vi "LM_I_11.15 - Copy.vi"   [LabVIEW 2012]
uses:
  <vilib>/NXT/Block Support/NXT_MessageMailbox.ctl
  <vilib>/NXT/Subs/MotorOutput.ctl
  <vilib>/NXT/Block Support/NXT_InputPort.ctl
  <vilib>/NXT/Block Support/NXT_TimerIndex.ctl
  <vilib>/NXT/Block Support/NXT_OutputPort.ctl
  <vilib>/NXT/Dual Mode Library/Advanced/NXTFlag_Assign.vi
  <vilib>/NXT/Dual Mode Library/BT/BlueTooth_Write_String.vi
types:
  T1 = typedef "MotorOutput.ctl" = u8
  T2 = typedef "NXT_MessageMailbox.ctl" = u8
  T3 = typedef "LVHSConnector.ctl" = refnum<class "BrickReference.lvclass">
  T4 = typedef "NXT_InputPort.ctl" = u32
  T5 = typedef "NXT_TimerIndex.ctl" = u8
  T6 = typedef "NXT_OutputPort.ctl" = u8
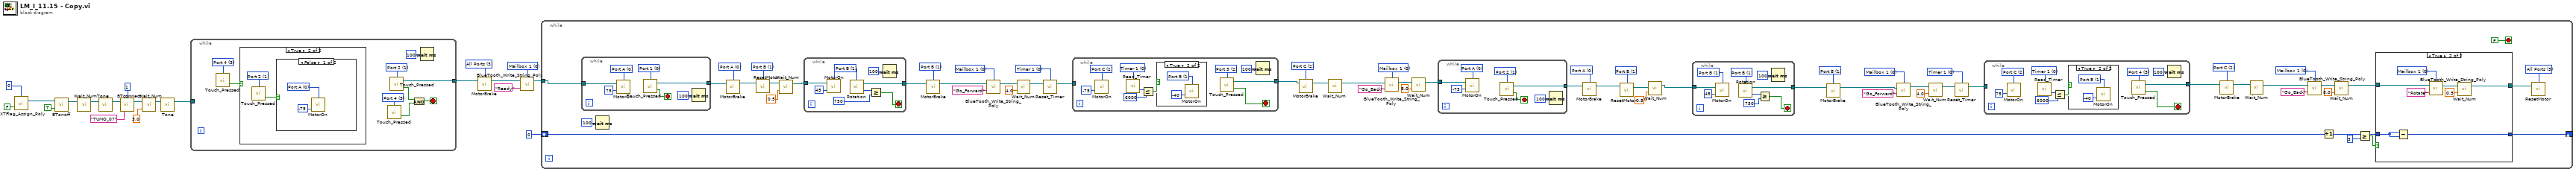
[diagram p0: block diagram]
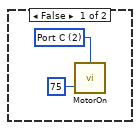
[diagram p2: hidden frame]
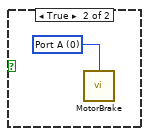
[diagram p3: hidden frame]
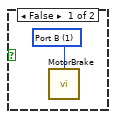
[diagram p4: hidden frame]
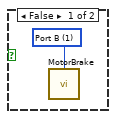
[diagram p6: hidden frame]
diagram:
  w7 = T1 3 items=["Port A"=0, "Port B"=1, "Port C"=2, "Ports A & B"=4, "Ports A & C"=5, "Ports B & C"=6, "All Ports"=3] ("Port (All Ports)")
  w8 = T2 0 items=["Mailbox 1", "Mailbox 2", "Mailbox 3", "Mailbox 4", "Mailbox 5", "Mailbox 6", "Mailbox 7", "Mailbox 8", "Mailbox 9", "Mailbox 10"] ("Mailbox")
  n1 = call-poly <vilib>:"NXTFlag_Assign_Poly.vi"("Flag State"=FALSE, "NXT/EV3 Flag Number"=i8 0) -> ("NXT/EV3"=w3:T3)  [unwired: 2 in]
  n2 = call <vilib>:"BTonoff.vi"("On/Off"=TRUE, "NXT/EV3"=w3) -> ("NXT/EV3"=w13:T3)  [unwired: 1 in, 1 out]
  n3 = call <vilib>:"Wait_Num.vi"("NXT/EV3"=w13) -> ("NXT/EV3"=w12:T3)  [unwired: 3 in]
  n4 = call <vilib>:"Tone.vi"("NXT/EV3"=w12) -> ("NXT/EV3"=w11:T3)  [unwired: 3 in]
  n5 = call <vilib>:"BTconnect.vi"("Partner Name"="TUMO_07", "NXT/EV3"=w11, "Connection"=u8 1) -> ("NXT/EV3"=w19:T3)  [unwired: 1 out]
  n6 = call <vilib>:"Wait_Num.vi"("Time (1 sec)"=sgl 3.0, "NXT/EV3"=w19) -> ("NXT/EV3"=w14:T3)  [unwired: 2 in]
  n7 = call <vilib>:"Tone.vi"("NXT/EV3"=w14) -> ("NXT/EV3"=w10:T3)  [unwired: 3 in]
  n8 = while {
    tunnel: w10 -> [_]
    tunnel: [w21] -> w5
    stop <- w25 stop-if-true
    w22 = T4 3 items=["Port 1", "Port 2", "Port 3", "Port 4"] ("Port (Port 1)")
    w27 = T4 3 items=["Port 1", "Port 2", "Port 3", "Port 4"] ("Port (Port 1)")
    w29 = T4 1 items=["Port 1", "Port 2", "Port 3", "Port 4"] ("Port (Port 1)")
    n9 = call <vilib>:"Touch_Pressed.vi"("Port (Port 1)"=w22) -> ("Yes / No"=w23:bool)  [unwired: 2 in, 1 out]
    n10 = case shown="True" w23 {
      frame False {
        w30 = T1 2 items=["Port A"=0, "Port B"=1, "Port C"=2, "Ports A & B"=4, "Ports A & C"=5, "Ports B & C"=6, "All Ports"=3] ("Output Port (All Ports)")
        n11 = call <vilib>:"MotorOn.vi"("Power (75)"=75, "Output Port (All Ports)"=w30) -> ()  [unwired: 2 in, 1 out]
      }
      frame True {
        w33 = T4 1 items=["Port 1", "Port 2", "Port 3", "Port 4"] ("Port (Port 1)")
        n12 = call <vilib>:"Touch_Pressed.vi"("Port (Port 1)"=w33) -> ("Yes / No"=w32:bool)  [unwired: 2 in, 1 out]
        n13 = case shown="False" w32 {
          frame False {
            w34 = T1 0 items=["Port A"=0, "Port B"=1, "Port C"=2, "Ports A & B"=4, "Ports A & C"=5, "Ports B & C"=6, "All Ports"=3] ("Output Port (All Ports)")
            n14 = call <vilib>:"MotorOn.vi"("Power (75)"=-75, "Output Port (All Ports)"=w34) -> ()  [unwired: 2 in, 1 out]
          }
          frame True {
            w36 = T1 0 items=["Port A"=0, "Port B"=1, "Port C"=2, "Ports A & B"=4, "Ports A & C"=5, "Ports B & C"=6, "All Ports"=3] ("Output Port (All Ports)")
            n15 = call <vilib>:"MotorBrake.vi"("Port (All Ports)"=w36) -> ()  [unwired: 3 in, 1 out]
          }
        }
      }
    }
    n16 = call <vilib>:"Touch_Pressed.vi"("Port (Port 1)"=w27) -> ("Yes / No"=w26:bool)  [unwired: 2 in, 1 out]
    n17 = call <vilib>:"Touch_Pressed.vi"("Port (Port 1)"=w29) -> ("Yes / No"=w28:bool, "NXT/EV3"=w21:T3)  [unwired: 2 in]
    n18 = And(x=w28, y=w26) -> (x .and. y?=w25:bool)
    n19 = Wait (ms)(milliseconds to wait=u32 100) -> ()  [unwired: 1 out]
  }
  n20 = call <vilib>:"MotorBrake.vi"("NXT/EV3"=w5, "Port (All Ports)"=w7) -> ("NXT/EV3"=w6:T3)  [unwired: 2 in]
  n21 = call-poly <vilib>:"BlueTooth_Write_String_Poly.vi"("Message"="Ready", "NXT/EV3"=w6, "Mailbox"=w8) -> ("NXT/EV3"=w4:T3)  [unwired: 1 in]
  n22 = while {
    shift-right: [w53] -> _
    shift-left: u32 0 ("milliseconds to wait") -> [w52]
    tunnel: w4 -> [w51]
    stop <- FALSE stop-if-true
    w37 = T1 3 items=["Port A"=0, "Port B"=1, "Port C"=2, "Ports A & B"=4, "Ports A & C"=5, "Ports B & C"=6, "All Ports"=3] ("Port (All Ports)")
    w43 = T5 0 items=["Timer 1", "Timer 2", "Timer 3"] ("Timer (Timer 1)")
    w47 = T5 0 items=["Timer 1", "Timer 2", "Timer 3"] ("Timer (Timer 1)")
    w91 = T1 1 items=["Port A"=0, "Port B"=1, "Port C"=2, "Ports A & B"=4, "Ports A & C"=5, "Ports B & C"=6, "All Ports"=3] ("Port (All Ports)")
    w90 = T1 1 items=["Port A"=0, "Port B"=1, "Port C"=2, "Ports A & B"=4, "Ports A & C"=5, "Ports B & C"=6, "All Ports"=3] ("Port (All Ports)")
    w76 = T2 0 items=["Mailbox 1", "Mailbox 2", "Mailbox 3", "Mailbox 4", "Mailbox 5", "Mailbox 6", "Mailbox 7", "Mailbox 8", "Mailbox 9", "Mailbox 10"] ("Mailbox")
    w74 = T2 0 items=["Mailbox 1", "Mailbox 2", "Mailbox 3", "Mailbox 4", "Mailbox 5", "Mailbox 6", "Mailbox 7", "Mailbox 8", "Mailbox 9", "Mailbox 10"] ("Mailbox")
    w69 = T2 0 items=["Mailbox 1", "Mailbox 2", "Mailbox 3", "Mailbox 4", "Mailbox 5", "Mailbox 6", "Mailbox 7", "Mailbox 8", "Mailbox 9", "Mailbox 10"] ("Mailbox")
    w67 = T1 2 items=["Port A"=0, "Port B"=1, "Port C"=2, "Ports A & B"=4, "Ports A & C"=5, "Ports B & C"=6, "All Ports"=3] ("Port (All Ports)")
    w65 = T1 0 items=["Port A"=0, "Port B"=1, "Port C"=2, "Ports A & B"=4, "Ports A & C"=5, "Ports B & C"=6, "All Ports"=3] ("Port (All Ports)")
    w64 = T1 2 items=["Port A"=0, "Port B"=1, "Port C"=2, "Ports A & B"=4, "Ports A & C"=5, "Ports B & C"=6, "All Ports"=3] ("Port (All Ports)")
    w61 = T1 1 items=["Port A"=0, "Port B"=1, "Port C"=2, "Ports A & B"=4, "Ports A & C"=5, "Ports B & C"=6, "All Ports"=3] ("Port (All Ports)")
    w60 = T1 0 items=["Port A"=0, "Port B"=1, "Port C"=2, "Ports A & B"=4, "Ports A & C"=5, "Ports B & C"=6, "All Ports"=3] ("Port (All Ports)")
    w57 = T2 0 items=["Mailbox 1", "Mailbox 2", "Mailbox 3", "Mailbox 4", "Mailbox 5", "Mailbox 6", "Mailbox 7", "Mailbox 8", "Mailbox 9", "Mailbox 10"] ("Mailbox")
    w55 = T1 1 items=["Port A"=0, "Port B"=1, "Port C"=2, "Ports A & B"=4, "Ports A & C"=5, "Ports B & C"=6, "All Ports"=3] ("Port (All Ports)")
    n23 = while {
      tunnel: [w160] -> w59
      tunnel: w51 -> [w159]
      stop <- w161 stop-if-true
      w162 = T4 0 items=["Port 1", "Port 2", "Port 3", "Port 4"] ("Port (Port 1)")
      w165 = T1 0 items=["Port A"=0, "Port B"=1, "Port C"=2, "Ports A & B"=4, "Ports A & C"=5, "Ports B & C"=6, "All Ports"=3] ("Output Port (All Ports)")
      n24 = call <vilib>:"MotorOn.vi"("Power (75)"=75, "NXT/EV3"=w159, "Output Port (All Ports)"=w165) -> ()  [unwired: 1 in, 1 out]
      n25 = call <vilib>:"Touch_Pressed.vi"("Port (Port 1)"=w162) -> ("Yes / No"=w161:bool, "NXT/EV3"=w160:T3)  [unwired: 2 in]
      n26 = Wait (ms)(milliseconds to wait=u32 100) -> ()  [unwired: 1 out]
    }
    n27 = Wait (ms)(milliseconds to wait=u32 100) -> ()  [unwired: 1 out]
    n28 = call <vilib>:"MotorBrake.vi"("NXT/EV3"=w59, "Port (All Ports)"=w60) -> ("NXT/EV3"=w58:T3)  [unwired: 2 in]
    n29 = call <vilib>:"ResetMotor.vi"("NXT/EV3"=w58, "Port (All Ports)"=w55) -> ("NXT/EV3"=w87:T3)  [unwired: 2 in]
    n30 = call <vilib>:"Wait_Num.vi"("Time (1 sec)"=sgl 0.5, "NXT/EV3"=w87) -> ("NXT/EV3"=w88:T3)  [unwired: 2 in]
    n31 = while {
      tunnel: w88 -> [w158]
      tunnel: [w152] -> w62
      stop <- w154 stop-if-true
      w156 = T1 1 items=["Port A"=0, "Port B"=1, "Port C"=2, "Ports A & B"=4, "Ports A & C"=5, "Ports B & C"=6, "All Ports"=3] ("Output Port (All Ports)")
      n32 = call <vilib>:"MotorOn.vi"("Power (75)"=45, "NXT/EV3"=w158, "Output Port (All Ports)"=w156) -> ()  [unwired: 1 in, 1 out]
      n33 = call <vilib>:"Rotation.vi"("Port (Port A)"=w156) -> ("Angle of Rotation"=w155:i32, "NXT/EV3"=w152:T3)  [unwired: 2 in]
      n34 = Greater Or Equal?(x=w155, y=750) -> (x >= y?=w154:bool)
      n35 = Wait (ms)(milliseconds to wait=u32 100) -> ()  [unwired: 1 out]
    }
    n36 = call <vilib>:"MotorBrake.vi"("NXT/EV3"=w62, "Port (All Ports)"=w61) -> ("NXT/EV3"=w63:T3)  [unwired: 2 in]
    n37 = call-poly <vilib>:"BlueTooth_Write_String_Poly.vi"("Message"="Go_Forward", "NXT/EV3"=w63, "Mailbox"=w57) -> ("NXT/EV3"=w50:T3)  [unwired: 1 in]
    n38 = call <vilib>:"Wait_Num.vi"("Time (1 sec)"=sgl 4.0, "NXT/EV3"=w50) -> ("NXT/EV3"=w48:T3)  [unwired: 2 in]
    n39 = call <vilib>:"Reset_Timer.vi"("NXT/EV3"=w48, "Timer (Timer 1)"=w47) -> ("NXT/EV3"=w46:T3)  [unwired: 2 in]
    n40 = while {
      tunnel: w46 -> [_]
      tunnel: [w138] -> w45
      stop <- w147 stop-if-true
      w139 = T5 0 items=["Timer 1", "Timer 2", "Timer 3"] ("Timer (Timer 1)")
      w144 = T1 2 items=["Port A"=0, "Port B"=1, "Port C"=2, "Ports A & B"=4, "Ports A & C"=5, "Ports B & C"=6, "All Ports"=3] ("Output Port (All Ports)")
      w146 = T4 2 items=["Port 1", "Port 2", "Port 3", "Port 4"] ("Port (Port 1)")
      n41 = call <vilib>:"MotorOn.vi"("Power (75)"=-75, "Output Port (All Ports)"=w144) -> ()  [unwired: 2 in, 1 out]
      n42 = call <vilib>:"Read_Timer.vi"("Timer (Timer 1)"=w139) -> ("Value (msec)"=w142:u32)  [unwired: 2 in, 1 out]
      n43 = Less Or Equal?(x=w142, y=u32 6000) -> (x <= y?=w140:bool)
      n44 = case shown="True" w140 {
        frame False {
          w148 = T1 1 items=["Port A"=0, "Port B"=1, "Port C"=2, "Ports A & B"=4, "Ports A & C"=5, "Ports B & C"=6, "All Ports"=3] ("Port (All Ports)")
          n45 = call <vilib>:"MotorBrake.vi"("Port (All Ports)"=w148) -> ()  [unwired: 3 in, 1 out]
        }
        frame True {
          w149 = T1 1 items=["Port A"=0, "Port B"=1, "Port C"=2, "Ports A & B"=4, "Ports A & C"=5, "Ports B & C"=6, "All Ports"=3] ("Output Port (All Ports)")
          n46 = call <vilib>:"MotorOn.vi"("Power (75)"=-40, "Output Port (All Ports)"=w149) -> ()  [unwired: 2 in, 1 out]
        }
      }
      n47 = call <vilib>:"Touch_Pressed.vi"("Port (Port 1)"=w146) -> ("Yes / No"=w147:bool, "NXT/EV3"=w138:T3)  [unwired: 2 in]
      n48 = Wait (ms)(milliseconds to wait=u32 100) -> ()  [unwired: 1 out]
    }
    n49 = call <vilib>:"MotorBrake.vi"("NXT/EV3"=w45, "Port (All Ports)"=w64) -> ("NXT/EV3"=w83:T3)  [unwired: 2 in]
    n50 = call <vilib>:"Wait_Num.vi"("NXT/EV3"=w83) -> ("NXT/EV3"=w84:T3)  [unwired: 3 in]
    n51 = call-poly <vilib>:"BlueTooth_Write_String_Poly.vi"("Message"="Go_Back", "NXT/EV3"=w84, "Mailbox"=w69) -> ("NXT/EV3"=w70:T3)  [unwired: 1 in]
    n52 = call <vilib>:"Wait_Num.vi"("Time (1 sec)"=sgl 8.0, "NXT/EV3"=w70) -> ("NXT/EV3"=w72:T3)  [unwired: 2 in]
    n53 = while {
      tunnel: [w132] -> w66
      tunnel: w72 -> [w131]
      stop <- w133 stop-if-true
      w134 = T4 1 items=["Port 1", "Port 2", "Port 3", "Port 4"] ("Port (Port 1)")
      w137 = T1 0 items=["Port A"=0, "Port B"=1, "Port C"=2, "Ports A & B"=4, "Ports A & C"=5, "Ports B & C"=6, "All Ports"=3] ("Output Port (All Ports)")
      n54 = call <vilib>:"MotorOn.vi"("Power (75)"=-75, "NXT/EV3"=w131, "Output Port (All Ports)"=w137) -> ()  [unwired: 1 in, 1 out]
      n55 = call <vilib>:"Touch_Pressed.vi"("Port (Port 1)"=w134) -> ("Yes / No"=w133:bool, "NXT/EV3"=w132:T3)  [unwired: 2 in]
      n56 = Wait (ms)(milliseconds to wait=u32 100) -> ()  [unwired: 1 out]
    }
    n57 = call <vilib>:"MotorBrake.vi"("NXT/EV3"=w66, "Port (All Ports)"=w65) -> ("NXT/EV3"=w95:T3)  [unwired: 2 in]
    n58 = call <vilib>:"ResetMotor.vi"("NXT/EV3"=w95, "Port (All Ports)"=w90) -> ("NXT/EV3"=w96:T3)  [unwired: 2 in]
    n59 = call <vilib>:"Wait_Num.vi"("Time (1 sec)"=sgl 0.5, "NXT/EV3"=w96) -> ("NXT/EV3"=w97:T3)  [unwired: 2 in]
    n60 = while {
      tunnel: [w116] -> w92
      tunnel: w97 -> [w113]
      stop <- w118 stop-if-true
      w114 = T6 1 items=["Port A", "Port B", "Port C", "Port D"] ("Port (Port A)")
      w115 = T1 1 items=["Port A"=0, "Port B"=1, "Port C"=2, "Ports A & B"=4, "Ports A & C"=5, "Ports B & C"=6, "All Ports"=3] ("Output Port (All Ports)")
      n61 = call <vilib>:"MotorOn.vi"("Power (75)"=45, "NXT/EV3"=w113, "Output Port (All Ports)"=w115) -> ()  [unwired: 1 in, 1 out]
      n62 = call <vilib>:"Rotation.vi"("Port (Port A)"=w114) -> ("Angle of Rotation"=w119:i32, "NXT/EV3"=w116:T3)  [unwired: 2 in]
      n63 = Greater Or Equal?(x=w119, y=750) -> (x >= y?=w118:bool)
      n64 = Wait (ms)(milliseconds to wait=u32 100) -> ()  [unwired: 1 out]
    }
    n65 = call <vilib>:"MotorBrake.vi"("NXT/EV3"=w92, "Port (All Ports)"=w91) -> ("NXT/EV3"=w94:T3)  [unwired: 2 in]
    n66 = call-poly <vilib>:"BlueTooth_Write_String_Poly.vi"("Message"="Go_Forward", "NXT/EV3"=w94, "Mailbox"=w74) -> ("NXT/EV3"=w40:T3)  [unwired: 1 in]
    n67 = call <vilib>:"Wait_Num.vi"("Time (1 sec)"=sgl 4.0, "NXT/EV3"=w40) -> ("NXT/EV3"=w42:T3)  [unwired: 2 in]
    n68 = call <vilib>:"Reset_Timer.vi"("NXT/EV3"=w42, "Timer (Timer 1)"=w43) -> ("NXT/EV3"=w44:T3)  [unwired: 2 in]
    n69 = while {
      tunnel: w44 -> [_]
      tunnel: [w99] -> w39
      stop <- w108 stop-if-true
      w100 = T5 0 items=["Timer 1", "Timer 2", "Timer 3"] ("Timer (Timer 1)")
      w105 = T1 2 items=["Port A"=0, "Port B"=1, "Port C"=2, "Ports A & B"=4, "Ports A & C"=5, "Ports B & C"=6, "All Ports"=3] ("Output Port (All Ports)")
      w107 = T4 3 items=["Port 1", "Port 2", "Port 3", "Port 4"] ("Port (Port 1)")
      n70 = call <vilib>:"MotorOn.vi"("Power (75)"=75, "Output Port (All Ports)"=w105) -> ()  [unwired: 2 in, 1 out]
      n71 = call <vilib>:"Read_Timer.vi"("Timer (Timer 1)"=w100) -> ("Value (msec)"=w103:u32)  [unwired: 2 in, 1 out]
      n72 = Less Or Equal?(x=w103, y=u32 6000) -> (x <= y?=w101:bool)
      n73 = case shown="True" w101 {
        frame False {
          w109 = T1 1 items=["Port A"=0, "Port B"=1, "Port C"=2, "Ports A & B"=4, "Ports A & C"=5, "Ports B & C"=6, "All Ports"=3] ("Port (All Ports)")
          n74 = call <vilib>:"MotorBrake.vi"("Port (All Ports)"=w109) -> ()  [unwired: 3 in, 1 out]
        }
        frame True {
          w110 = T1 1 items=["Port A"=0, "Port B"=1, "Port C"=2, "Ports A & B"=4, "Ports A & C"=5, "Ports B & C"=6, "All Ports"=3] ("Output Port (All Ports)")
          n75 = call <vilib>:"MotorOn.vi"("Power (75)"=-40, "Output Port (All Ports)"=w110) -> ()  [unwired: 2 in, 1 out]
        }
      }
      n76 = call <vilib>:"Touch_Pressed.vi"("Port (Port 1)"=w107) -> ("Yes / No"=w108:bool, "NXT/EV3"=w99:T3)  [unwired: 2 in]
      n77 = Wait (ms)(milliseconds to wait=u32 100) -> ()  [unwired: 1 out]
    }
    n78 = call <vilib>:"MotorBrake.vi"("NXT/EV3"=w39, "Port (All Ports)"=w67) -> ("NXT/EV3"=w85:T3)  [unwired: 2 in]
    n79 = call <vilib>:"Wait_Num.vi"("NXT/EV3"=w85) -> ("NXT/EV3"=w86:T3)  [unwired: 3 in]
    n80 = call-poly <vilib>:"BlueTooth_Write_String_Poly.vi"("Message"="Go_Back", "NXT/EV3"=w86, "Mailbox"=w76) -> ("NXT/EV3"=w77:T3)  [unwired: 1 in]
    n81 = Increment(x=w52) -> (x+1=w81:u32)
    n82 = call <vilib>:"Wait_Num.vi"("Time (1 sec)"=sgl 8.0, "NXT/EV3"=w77) -> ("NXT/EV3"=w82:T3)  [unwired: 2 in]
    n83 = Greater Or Equal?(x=w81, y=u32 3) -> (x >= y?=w80:bool)
    n84 = case shown="True" w80 {
      tunnel: w81 -> [w122 w130]
      tunnel: [w122 w124] -> w53
      tunnel: w82 -> [w121 w125]
      tunnel: [w121 w123] -> w38
      frame False {
      }
      frame True {
        w128 = T2 0 items=["Mailbox 1", "Mailbox 2", "Mailbox 3", "Mailbox 4", "Mailbox 5", "Mailbox 6", "Mailbox 7", "Mailbox 8", "Mailbox 9", "Mailbox 10"] ("Mailbox")
        n85 = Subtract(x=w130, y=w130) -> (x-y=w124:u32)
        n86 = call-poly <vilib>:"BlueTooth_Write_String_Poly.vi"("Message"="Rotate", "NXT/EV3"=w125, "Mailbox"=w128) -> ("NXT/EV3"=w127:T3)  [unwired: 1 in]
        n87 = call <vilib>:"Wait_Num.vi"("Time (1 sec)"=sgl 0.5, "NXT/EV3"=w127) -> ("NXT/EV3"=w123:T3)  [unwired: 2 in]
      }
    }
    n88 = call <vilib>:"ResetMotor.vi"("NXT/EV3"=w38, "Port (All Ports)"=w37) -> ()  [unwired: 2 in, 1 out]
  }
